vi "Select Path.vi"(6 "error in":errorcluster) -> (0 "error out":errorcluster, 1 "Save?":bool, 2 "selected path":path, 3 "Path":string)   [LabVIEW 2016, in "Data Saving.lvlib" / "Abstract Saver.lvclass"]
uses:
  Abstract Saver.lvclass
  Data Logger/PathFinder Type def.ctl
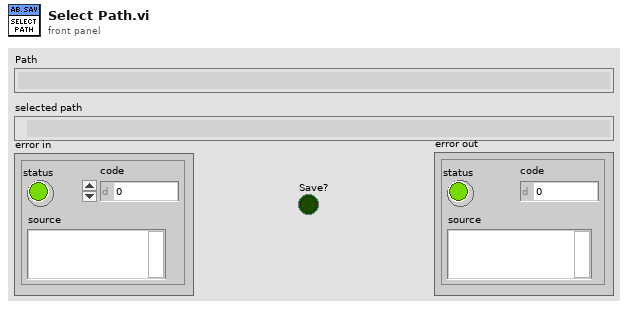
[diagram p1: front panel]
types:
  T1 = typedef "PathFinder Type def.ctl" = enum16{"Done", "Waiting"}
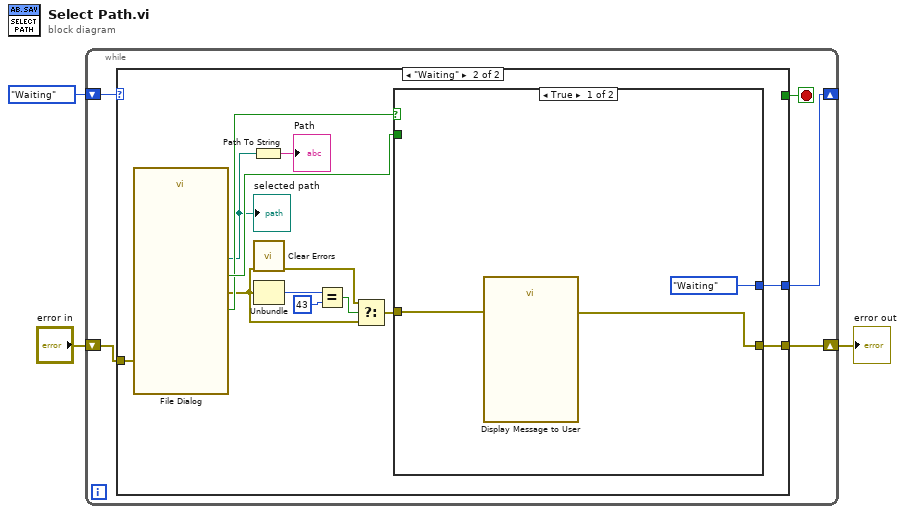
[diagram p0: block diagram]
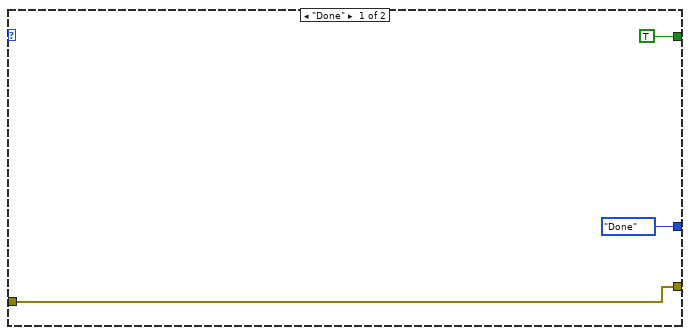
[diagram p2: hidden frame]
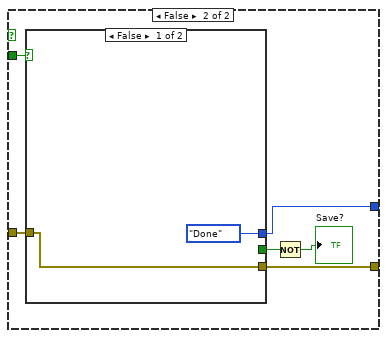
[diagram p3: hidden frame]
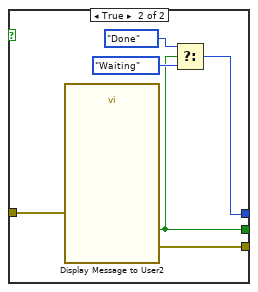
[diagram p4: hidden frame]
diagram:
  n1 = while {
    shift-right: [w6] -> _
    shift-left: PathFinder_Type_def."Waiting" -> [w8]
    shift-right: [w4] -> w1
    shift-left: "error in" -> [w5]
    stop <- w7 stop-if-true
    n2 = case shown="\"Waiting\"" w8 {
      tunnel: [TRUE _] -> w7
      tunnel: [PathFinder_Type_def."Done" w22] -> w6
      tunnel: w5 -> [w10 w19]
      tunnel: [w10 w18] -> w4
      frame "Done" {
      }
      frame "Waiting" {
        n3 = call "File Dialog"("error in"=w19) -> ("selected path"=w21:path, "exists"=w23:bool, "cancelled"=w24:bool, "error out"=w13:errorcluster)  [unwired: 11 in]
        "selected path" <- w21
        n4 = Path To String(path=w21) -> (string=→"Path":string)
        n5 = call <vilib>:"Clear Errors.vi"("error in (no error)"=w13) -> ("error out"=w14:errorcluster)  [unwired: 5 in, 1 out]
        n6 = Unbundle(w13) -> ("code"=w17:i32)  [unwired: 2 out]
        n7 = Equal?(x=w17, y=43) -> (x = y?=w15:bool)
        n8 = Select(t=w14, s=w15, f=w13) -> (s? t:f=w12:errorcluster)
        n9 = case shown="True" w23 {
          tunnel: w24 -> [_ w33]
          tunnel: [PathFinder_Type_def."Waiting" w32] -> w22
          tunnel: w12 -> [w26 w29]
          tunnel: [w25 w28] -> w18
          frame True {
            n10 = call "Display Message to User"("error in (no error)"=w26) -> ("error out"=w25:errorcluster)  [unwired: 9 in, 1 out]
          }
          frame False {
            n11 = case shown="False" w33 {
              tunnel: [PathFinder_Type_def."Done" w39] -> w32
              tunnel: [_ w38] -> w31
              tunnel: w29 -> [w34 w37]
              tunnel: [w34 w36] -> w28
              frame False {
              }
              frame True {
                n12 = call "Display Message to User2"("error in (no error)"=w37) -> ("error out"=w36:errorcluster, "Do Not Save"=w38:bool)  [unwired: 9 in]
                n13 = Select(t=PathFinder_Type_def."Done", s=w38, f=PathFinder_Type_def."Waiting") -> (s? t:f=w39:T1)
              }
            }
            n14 = Not(x=w31) -> (.not. x?=→"Save?":bool)
          }
        }
      }
    }
  }
  "error out" <- w1
